vi "Get Index.vi"(11 "File Path Control":path) -> (2 "DBL number":dbl, 3 "Index":i32)   [LabVIEW 2016]
panel:
  out "match + rest of string":string
  out "match substring":string
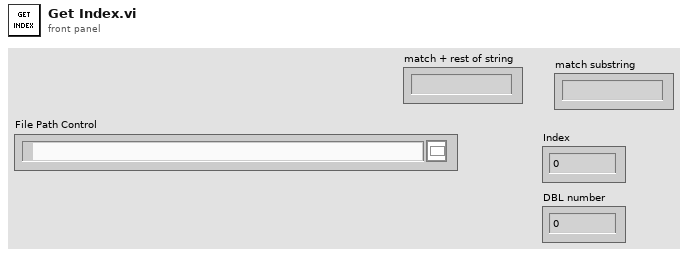
[diagram p1: front panel]
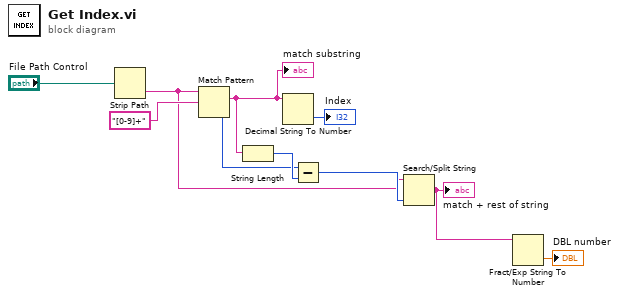
[diagram p0: block diagram]
diagram:
  n1 = Strip Path(path="File Path Control") -> (name=w3:string)  [unwired: 1 out]
  n2 = Match Pattern(string=w3, regular expression="[0-9]+") -> (match substring=w7:string, offset past match=w5:i32)  [unwired: 1 in, 2 out]
  "match substring" <- w7
  n3 = String Length(string=w7) -> (length=w6:i32)
  n4 = Decimal String To Number(string=w7) -> (number=→"Index":i32)  [unwired: 2 in, 1 out]
  n5 = Subtract(x=w5, y=w6) -> (x-y=w4:i32)
  n6 = Search/Split String(string=w3, offset (0)=w4) -> (match + rest of string=w2:string)  [unwired: 1 in, 2 out]
  "match + rest of string" <- w2
  n7 = Fract/Exp String To Number(string=w2) -> (number=→"DBL number":dbl)  [unwired: 3 in, 1 out]
